vi "Get Abbreviated Date.vi"() -> (2 "Abrreviated Data":string)   [LabVIEW 2018]
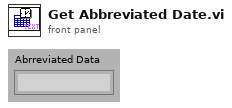
[diagram p1: front panel]
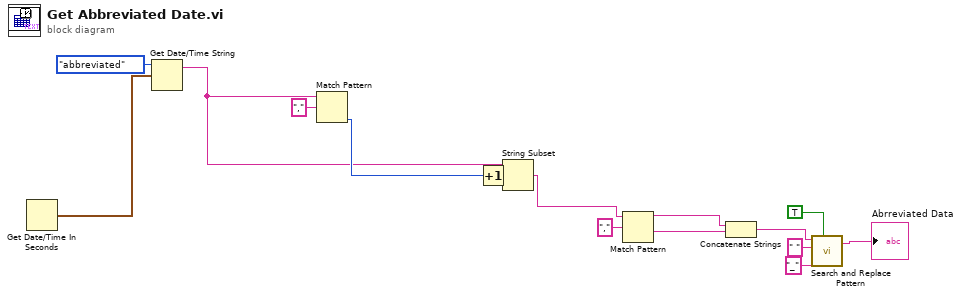
[diagram p0: block diagram]
diagram:
  n1 = Get Date/Time In Seconds() -> (seconds since 1Jan1904=w2:timestamp)
  n2 = Get Date/Time String(date format (0)=enum16{"short", "long", "abbreviated"}."abbreviated", seconds (now)=w2) -> (date string=w12:string)  [unwired: 1 in, 1 out]
  n3 = Match Pattern(string=w12, regular expression=",") -> (offset past match=w13:i32)  [unwired: 1 in, 3 out]
  n4 = Increment(x=w13) -> (x+1=w11:i32)
  n5 = String Subset(string=w12, offset (0)=w11) -> (substring=w9:string)  [unwired: 1 in]
  n6 = Match Pattern(string=w9, regular expression=",") -> (before substring=w8:string, after substring=w7:string)  [unwired: 1 in, 2 out]
  n7 = Concatenate Strings(w8, w7) -> (w6:string)
  n8 = call <vilib>:"Search and Replace Pattern.vi"("string"=w6, "regular expression (\"\")"=" " ("regular expression (\"\")"), "replace string (\"\")"="_" ("replace string (\"\")"), "replace all? (F)"=TRUE) -> ("result string"=→"Abrreviated Data":string)  [unwired: 1 in, 1 out]
